vi "tmp1bindata to XD arr.vi"(4 "numtype in":string, 6 "arrdims":i32[](array[numeric]), 7 "type in":i64, 8 "error in (no error)":errorcluster, 9 "start":i32=-1, 10 "nofbytes":i32=-1, 11 "bindata in":u8[](array[numeric])) -> (0 "error out":errorcluster, 1 "numarray 3D":i64[][][](array[numeric]), 2 "numarray 2D":i64[][](array[numeric]), 3 "numarray 1D":i64[](array[numeric]), 5 "x-y*floor(x/y)":i32)   [LabVIEW 2018]
uses:
  17a11fa0-ca30-411f-bf81-781a9d4b2792.vi
  <vilib>/Utility/error.llb/Error Cluster From Error Code.vi
  <vilib>/ErrorRing/Error Ring.xnode
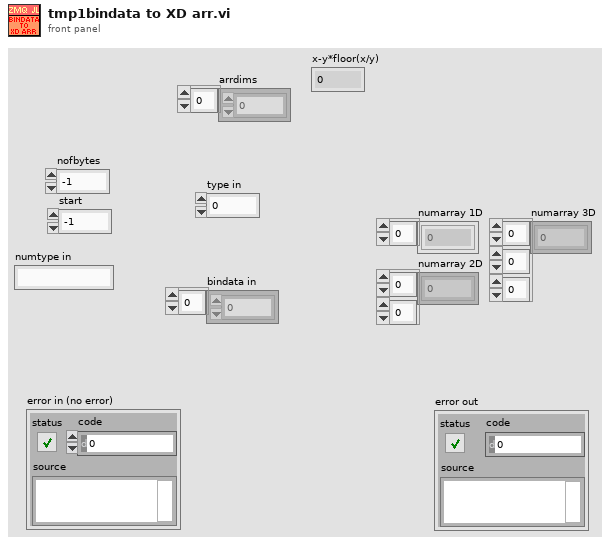
[diagram p1: front panel]
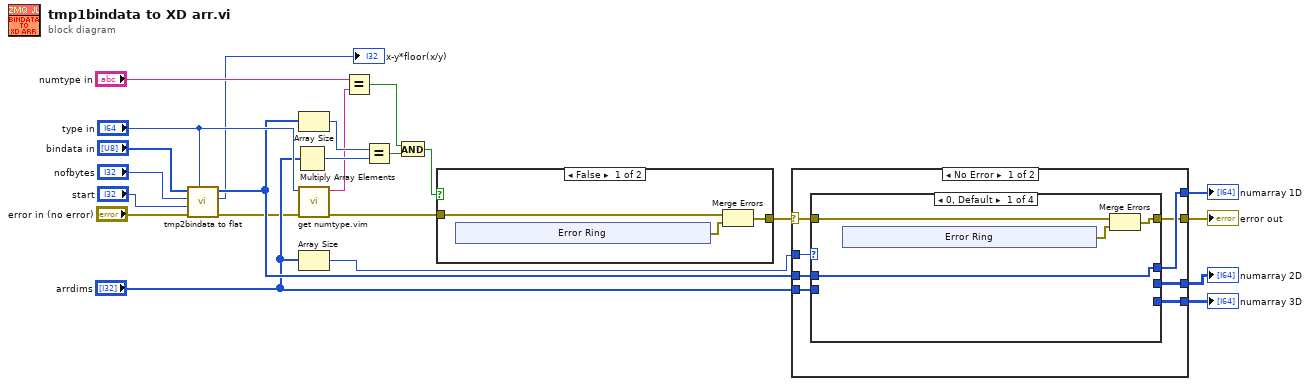
[diagram p0: block diagram]
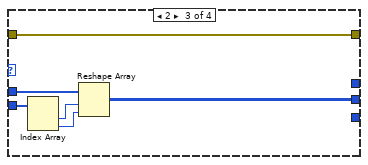
[diagram p3: hidden frame]
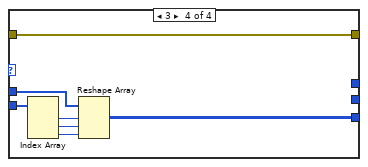
[diagram p4: hidden frame]
diagram:
  n1 = call "tmp2bindata to flat.vi"("type in"="type in", "error in (no error)"="error in (no error)", "start"="start", "nofbytes"="nofbytes", "bindata in"="bindata in") -> ("error out"=w2:errorcluster, "x-y*floor(x/y)"=→"x-y*floor(x/y)":i32, "numarray out"=w11:i64[])  [unwired: 4 in]
  n2 = Multiply Array Elements(1:"arrdims") -> (0:w19:i32)
  n3 = Array Size(array=w11) -> (size(s)=w18:i32)
  n4 = call "get numtype.vim"("error in (no error)"=w2, "type in"="type in") -> ("error out"=w16:errorcluster, "numtype out"=w14:string)  [unwired: 8 in]
  n5 = Array Size(array="arrdims") -> (size(s)=w10:i32)
  n6 = Equal?(x="numtype in", y=w14) -> (x = y?=w20:bool)
  n7 = Equal?(x=w18, y=w19) -> (x = y?=w17:bool)
  n8 = And(x=w20, y=w17) -> (x .and. y?=w21:bool)
  n9 = case shown="False" w21 {
    tunnel: [w25 w32] -> w13
    tunnel: w16 -> [w26 w32]
    frame False {
      n10 = xnode "Error Ring"() -> ("error out"=w24:errorcluster)
      n11 = Merge Errors(w26, w24) -> (w25:errorcluster)
    }
    frame True {
    }
  }
  n12 = case shown="No Error" w13 {
    selector: w13 -> [w34 w65]
    tunnel: [w33 w65] -> w12
    tunnel: w11 -> [w39 _]
    tunnel: w10 -> [w40 _]
    tunnel: [w38 _] -> w9
    tunnel: "arrdims" -> [w37 _]
    tunnel: [w36 _] -> w8
    tunnel: [w35 _] -> w7
    frame No Error {
      n13 = case shown="0, Default" w40 {
        tunnel: w39 -> [w41 w51 w55 w62]
        tunnel: [w41 w51 _ _] -> w38
        tunnel: w37 -> [_ _ w54 w61]
        tunnel: [_ _ w53 _] -> w36
        tunnel: [_ _ _ w60] -> w35
        tunnel: [w43 w50 w52 w58] -> w33
        tunnel: w34 -> [w44 w50 w52 w58]
        frame 0, Default {
          n14 = xnode "Error Ring"() -> ("error out"=w42:errorcluster)
          n15 = Merge Errors(w44, w42) -> (w43:errorcluster)
        }
        frame 1 {
        }
        frame 2 {
          n16 = Index Array(array=w54) -> (element #1=w56:i32, element #2=w57:i32)  [unwired: 2 in]
          n17 = Reshape Array(w55, w56, w57) -> (w53:i64[][])
        }
        frame 3 {
          n18 = Index Array(array=w61) -> (element #1=w63:i32, element #2=w64:i32, element #3=w59:i32)  [unwired: 3 in]
          n19 = Reshape Array(w62, w63, w64, w59) -> (w60:i64[][][])
        }
      }
    }
    frame Error {
    }
  }
  "error out" <- w12
  "numarray 1D" <- w9
  "numarray 2D" <- w8
  "numarray 3D" <- w7
